vi "Convert Overrides.vi"(10 "Cluster":cluster{dbl[], bool[]}, 11 "Velocity (fps)":dbl) -> (3 "Overrides":T1=[{"Count"="1", "Angular Override"=15.0, "Enabled?"=FALSE, "Velocity Override"=6.0, "Angle Override"=6.0}] {"Angle Override" step=5.0; "Velocity Override" step=5.0; "Angular Override" step=5.0})   [LabVIEW 2025]
uses:
  Types/Overrides.ctl
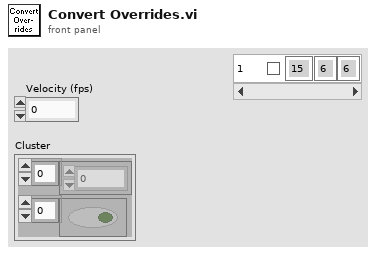
[diagram p1: front panel]
types:
  T1 = typedef "Overrides.ctl" = cluster{"Count":string, "Angular Override":dbl, "Enabled?":bool, "Velocity Override":dbl, "Angle Override":dbl}[]
  T2 = cluster{string, "Angular Multiplier":dbl, "1":bool, "Velocity (fps)":dbl, "Velocity (fps)":dbl}
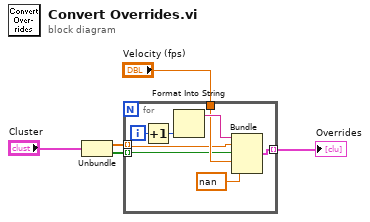
[diagram p0: block diagram]
diagram:
  n1 = Unbundle("Cluster") -> (w3:dbl[], w2:bool[])
  n2 = for {
    tunnel: [w13] -> w1 mode=indexing
    tunnel: "Velocity (fps)" -> [w10]
    tunnel: w3 -> [w9] mode=indexing
    tunnel: w2 -> [w8] mode=indexing
    i -> [w12]
    n3 = Increment(x=w12) -> (x+1=w7:i32)
    n4 = Format Into String(w7) -> (resulting string=w11:string)  [unwired: 3 in, 1 out]
    n5 = Bundle(w11, "Angular Multiplier"=w9, "1"=w8, "Velocity (fps)"=w10, "Velocity (fps)"=nan) -> (w13:T2)  [unwired: 1 in]
  }
  "Overrides" <- w1
